vi "SEND CAN data.vi"() -> ()   [LabVIEW 2016]
doc: "This is a practical example of CAN_WRITE.\nFirst of all the selected channel will be initiatlized.\nOnce the initialisation is OK a timed while loop will be executed until CAN_WRITE will signal an error.\nSince CAN_WRITE is limited to eight bytes this example transmitts only 4 Bytes."
uses:
  CAN Communication.llb/TPCANHandle.ctl
  CAN Communication.llb/TPCANBaudrate.ctl
  CAN Communication.llb/CAN MSG Cluster.ctl
  CAN Communication.llb/TPCANParameter.ctl
  <vilib>/Platform/TimedLoop/XDataNode/timing_clust.ctl
  <vilib>/Platform/TimedLoop/XDataNode/nitl_modes.ctl
  <vilib>/Platform/TimedLoop/XDataNode/wakeup.ctl
  CAN Communication.llb/PCAN Get CHANNEL CONDITION.vi
  <vilib>/Platform/TimedLoop/XDataNode/XDataNode.xnode
  <vilib>/Platform/TimedLoop/XDataNode/XDNodeRunTimeDep.lvlib
panel:
  out "error out":errorcluster
  out "input cluster":T1 {"MSG type" format="%x"; "ID" format="%.0x"}
  in  "Release all channels first":bool=TRUE
  in  "TPCANBaudrate":T2
  in  "TPCANHandle":T3=enum."PCAN_USBBUS1  0x51"
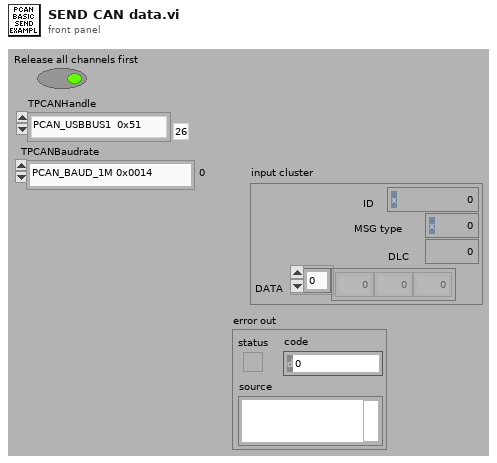
[diagram p1: front panel]
types:
  T1 = typedef "CAN MSG Cluster.ctl" = cluster{"ID":u32, "MSG type":u8, "DLC":u8, "DATA":u8[]}
  T2 = typedef "TPCANBaudrate.ctl" = enum16{"PCAN_BAUD_1M 0x0014", "PCAN_BAUD_800K 0x0016", "PCAN_BAUD_500K 0x001C", "PCAN_BAUD_250K 0x011C", "PCAN_BAUD_125K 0x031C", "PCAN_BAUD_100K 0x432F", "PCAN_BAUD_95K 0xC34E", "PCAN_BAUD_83K 0x852B", "PCAN_BAUD_50K 0x472F", "PCAN_BAUD_47K 0x1414", "PCAN_BAUD_33K 0x8B2F", "PCAN_BAUD_20K 0x532F", "PCAN_BAUD_10K 0x672F", "PCAN_BAUD_5K 0x7F7F", "User Baudrate"}
  T3 = typedef "TPCANHandle.ctl" = enum16{"PCAN_NONEBUS  0x000", "PCAN_ISABUS1  0x21", "PCAN_ISABUS2  0x22", "PCAN_ISABUS3  0x23", "PCAN_ISABUS4  0x24", "PCAN_ISABUS5  0x25", "PCAN_ISABUS6  0x26", "PCAN_ISABUS7  0x27", "PCAN_ISABUS8  0x28", "PCAN_DNGBUS1  0x31", "PCAN_PCIBUS1  0x41", "PCAN_PCIBUS1  0x42", "PCAN_PCIBUS1  0x43", "PCAN_PCIBUS1  0x44", "PCAN_PCIBUS1  0x45", "PCAN_PCIBUS1  0x46", "PCAN_PCIBUS1  0x47", "PCAN_PCIBUS1  0x48", "PCAN_PCIBUS1  0x409", "PCAN_PCIBUS1  0x40A", "PCAN_PCIBUS1  0x40B", "PCAN_PCIBUS1  0x40C", "PCAN_PCIBUS1  0x40D", "PCAN_PCIBUS1  0x40E", "PCAN_PCIBUS1  0x40F", "PCAN_PCIBUS1  0x410", "PCAN_USBBUS1  0x51", "PCAN_USBBUS2  0x52", "PCAN_USBBUS3  0x53", "PCAN_USBBUS4  0x54", "PCAN_USBBUS5  0x55", "PCAN_USBBUS6  0x56", "PCAN_USBBUS7  0x57", "PCAN_USBBUS8  0x58", "PCAN_USBBUS9  0x509", "PCAN_USBBUS10  0x50A", "PCAN_USBBUS11  0x50B", "PCAN_USBBUS12  0x50C", "PCAN_USBBUS13  0x50D", "PCAN_USBBUS14  0x50E", "PCAN_USBBUS15  0x50F", "PCAN_USBBUS16  0x510", "PCAN_PCCBUS1  0x61", "PCAN_PCCBUS2  0x62", "PCAN_LANBUS1  0x801", "PCAN_LANBUS2  0x802", "PCAN_LANBUS3  0x803", "PCAN_LANBUS4  0x804", "PCAN_LANBUS5  0x805", "PCAN_LANBUS6  0x806", "PCAN_LANBUS7  0x807", "PCAN_LANBUS8  0x808", "PCAN_LANBUS9  0x809", "PCAN_LANBUS10  0x80A", "PCAN_LANBUS11  0x80B", "PCAN_LANBUS12  0x80C", "PCAN_LANBUS13  0x80D", "PCAN_LANBUS14  0x80E", "PCAN_LANBUS15  0x80F", "PCAN_LANBUS16  0x810"}
  T4 = typedef "TPCANParameter.ctl" = enum8{"Not Available", "PCAN device number", "PCAN 5-volt power", "PCAN receive event", "PCAN message filter", "PCAN API version", "PCAN channel version", "PCAN busoff autoreset", "PCAN listen-only", "PCAN log location", "PCAN log status", "PCAN log configure", "PCAN log text", "PCAN channel condition", "PCAN hardware name", "PCAN_RECEIVE_STATUS", "PCAN_CONTROLLER_NUMBER", "PCAN_TRACE_LOCATION ", "PCAN_TRACE_STATUS", "PCAN_TRACE_SIZE", "PCAN_TRACE_CONFIGURE", "PCAN_CHANNEL_IDENTIFYING", "PCAN_CHANNEL_FEATURES", "PCAN_SPEED_ADAPTING", "PCAN_BITRATE_INFO", "PCAN_BITRATE_INFO_FD", "PCAN_BUSSPEED_NOMINAL", "PCAN_BUSSPEED_DATA", "PCAN_IP_ADDRESS", "PCAN_LAN_SERVICE_STATUS", "PCAN_ALLOW_STATUS_FRAMES", "PCAN_ALLOW_RTR_FRAMES", "PCAN_ALLOW_ERROR_FRAMES", "PCAN_INTERFRAME_DELAY", "PCAN_ACCEPTANCE_FILTER_11BIT", "PCAN_ACCEPTANCE_FILTER_29BIT", "PCAN_IO_DIGITAL_CONFIGURATION", "PCAN_IO_DIGITAL_VALUE", "PCAN_IO_DIGITAL_SET", "PCAN_IO_DIGITAL_CLEAR", "PCAN_IO_ANALOG_VALUE"}
  T5 = typedef "Channel Availability.ctl" = enum16{"PCAN_CHANNEL_UNAVAILABLE", "PCAN_CHANNEL_AVAILABLE", "PCAN_CHANNEL_OCCUPIED"}
  T6 = typedef "XDNodeRunTimeDep.lvlib/timing_clust.ctl" = cluster{"Expected End [f-1]":u64, "Actual End [f-1]":u64, "Finished Late? [f-1]":bool, "Expected End [i-1]":u64, "Actual End [i-1]":u64, "Finished Late? [i-1]":bool, "Expected Start [i]":u64, "Actual Start [i]":u64, "Expected Start [f]":u64, "Actual Start [f]":u64, "Source Name":string, "Structure Name":string, "Period":i64, "Deadline":i64, "Offset":i64, "Start":i64, "Priority":i32, "Timeout":i32, "Mode":T7, "Wakeup Reason":T8, "Error":errorcluster, "Source Type":string, "Secondary Source Type":string, "Global End Time":u64, "Global Start Time":u64, "Frame Duration":u64, "Iteration Duration":u64, "Assigned CPU":i32, "I/O Scan Engine Mode":u32}
  T7 = typedef "XDNodeRunTimeDep.lvlib/nitl_modes.ctl" = enum32{"No Change", "Process missed periods, maintain original phase", "Discard missed periods, maintain original phase", "Process missed periods, ignore original phase", "Discard missed periods, ignore original phase"}
  T8 = typedef "XDNodeRunTimeDep.lvlib/wakeup.ctl" = enum32{"Normal", "Aborted", "Asynchronous wakeup", "Timing source error", "Timed loop error", "Timeout"}
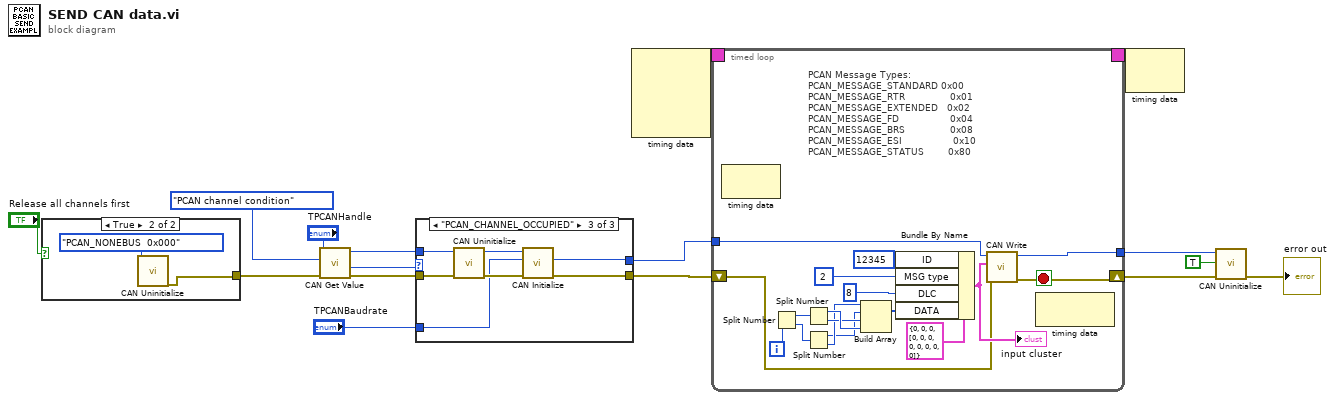
[diagram p0: block diagram]
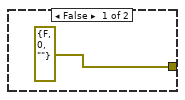
[diagram p2: hidden frame]
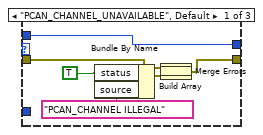
[diagram p3: hidden frame]
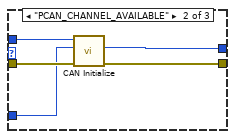
[diagram p4: hidden frame]
diagram:
  n1 = case shown="True" "Release all channels first" {
    tunnel: [errorcluster {"status"=FALSE, "code"=0, "source"=""} ("error out") w19] -> w10
    frame False {
    }
    frame True {
      n2 = call "CAN Uninitialize.vi"("TPCANHandle"=TPCANHandle."PCAN_NONEBUS  0x000" ("Channel")) -> ("error out"=w19:errorcluster)  [unwired: 8 in, 2 out]
    }
  }
  n3 = call-poly "CAN Get Value.vi"("error in (no error)"=w10, "TPCANParameter"=TPCANParameter."PCAN channel condition" ("Parameter"), "TPCANHandle"="TPCANHandle") -> ("error out"=w13:errorcluster, "Channel condition"=w12:T5, "TPCANHandle out"=w14:T3)  [unwired: 6 in]
  n4 = case shown="\"PCAN_CHANNEL_OCCUPIED\"" w12 {
    tunnel: [w25 w31 w35] -> w5
    tunnel: w14 -> [w26 w30 w37]
    tunnel: w13 -> [w24 w29 w38]
    tunnel: "TPCANBaudrate" -> [_ w27 w32]
    tunnel: [w26 w28 w34] -> w6
    frame "PCAN_CHANNEL_UNAVAILABLE", Default {
      n5 = Bundle By Name(cluster=w24, "status"=TRUE, "source"="PCAN_CHANNEL ILLEGAL") -> (w21:errorcluster)
      n6 = Build Array(w24, w21) -> (w20:errorcluster[])
      n7 = Merge Errors(w20) -> (w25:errorcluster)
    }
    frame "PCAN_CHANNEL_AVAILABLE" {
      n8 = call "CAN Initialize.vi"("error in (no error)"=w29, "TPCANBaudrate"=w27, "TPCANHandle"=w30) -> ("error out"=w31:errorcluster, "TPCANHandle_out"=w28:T3)  [unwired: 6 in, 1 out]
    }
    frame "PCAN_CHANNEL_OCCUPIED" {
      n9 = call "CAN Uninitialize.vi"("error in (no error)"=w38, "TPCANHandle"=w37) -> ("error out"=w36:errorcluster, "TPCANHandle out"=w33:T3)  [unwired: 7 in, 1 out]
      n10 = call "CAN Initialize.vi"("error in (no error)"=w36, "TPCANBaudrate"=w32, "TPCANHandle"=w33) -> ("error out"=w35:errorcluster, "TPCANHandle_out"=w34:T3)  [unwired: 6 in, 1 out]
    }
  }
  n11 = node-c288() -> (w8:T6)  [unwired: 4 in]
  n12 = timed-loop {
    timing: w8 -> [_]
    timing-out: [_] -> w7
    tunnel: w6 -> [w55]
    shift-right: [w42] -> w4
    shift-left: w5 -> [w43]
    tunnel: [w39] -> w2
    i -> [w51]
    stop <- w42 stop-if-true
    # "PCAN Message Types:\nPCAN_MESSAGE_STANDARD 0x00\nPCAN_MESSAGE_RTR               0x01\nPCAN_MESSAGE_EXTENDED   0x02\nPCAN_MESSAGE_FD                 0x04\nPCAN_MESSAGE_BRS               0x08\nPCAN_MESSAGE_ESI                 0x10\nPCAN_MESSAGE_STATUS        0x80"
    n13 = node-c288() -> ()  [unwired: 1 in, 1 out]
    n14 = Split Number(x=w51) -> (hi(x)=w49:u16, lo(x)=w50:u16)
    n15 = Split Number(x=w49) -> (hi(x)=w48:u8, lo(x)=w47:u8)
    n16 = Split Number(x=w50) -> (hi(x)=w44:u8, lo(x)=w45:u8)
    n17 = Build Array(w45, w44, w47, w48) -> (w46:u8[])
    n18 = Bundle By Name(cluster=T1 {"ID"=0, "MSG type"=0, "DLC"=0, "DATA"=[0, 0, 0, 0, 0, 0, 0, 0]} ("CAN_Message"), "ID"=u32 12345, "MSG type"=u8 2, "DLC"=i8 8 ("LEN"), "DATA"=w46) -> (w54:T1)
    "input cluster" <- w54
    n19 = call "CAN Write.vi"("error in (no error)"=w43, "CAN_Message"=w54, "TPCANHandle"=w55) -> ("error out"=w42:errorcluster, "TPCANHandle out"=w39:T3)  [unwired: 7 in]
    n20 = node-c288() -> ()  [unwired: 1 in, 1 out]
  }
  n21 = node-c288(w7) -> ()  [unwired: 1 out]
  n22 = call "CAN Uninitialize.vi"("error in (no error)"=w4, "Ignore input error"=TRUE, "TPCANHandle"=w2) -> ("error out"=→"error out":errorcluster)  [unwired: 6 in, 2 out]
